vi "Write Sweep Rate (No Objects).vi"(8 "error in (no error)":errorcluster, 10 "rate":dbl[unit] caption="Rate", 11 "Cluster In":T4={"Field"=0.0, "Rate"=0.0, "Status"={"Sweeping"=FALSE, "Clamped"=FALSE, "Hold"=FALSE, "At Rest"=FALSE, "Quench"=FALSE, "Persistent Mode"=FALSE, "Switch Heater"=FALSE}, "ILM Shut Down?"=FALSE, "IO Info"={"Address"={"Com Port"=1, "ISOBUS Address"=2, "GPIB Address"=24, "Communication"=enum."ISOBUS"}, "Version"=enum."IPS"}, "IO Info (Level Meter)"={"Address"={"Com Port"=1, "ISOBUS Address"=5, "GPIB Address"=24, "Communication"=enum."ISOBUS"}, "ILM Name"="", "Display Channel"=[]}, "Training?"=FALSE, "Training Field and Speed Cluster"={"Training Field"=[0.0, 4.108, 5.78, 8.001], "Training Speed"=[0.0057, 0.0022833333333333334, 0.0011333333333333334, 0.0011333333333333334]}}) -> (0 "error out":errorcluster, 3 "Cluster Out":T4={"Field"=0.0, "Rate"=0.0, "Status"={"Sweeping"=FALSE, "Clamped"=FALSE, "Hold"=FALSE, "At Rest"=FALSE, "Quench"=FALSE, "Persistent Mode"=FALSE, "Switch Heater"=FALSE}, "ILM Shut Down?"=FALSE, "IO Info"={"Address"={"Com Port"=1, "ISOBUS Address"=2, "GPIB Address"=24, "Communication"=enum."ISOBUS"}, "Version"=enum."IPS"}, "IO Info (Level Meter)"={"Address"={"Com Port"=1, "ISOBUS Address"=5, "GPIB Address"=24, "Communication"=enum."ISOBUS"}, "ILM Name"="", "Display Channel"=[]}, "Training?"=FALSE, "Training Field and Speed Cluster"={"Training Field"=[0.0, 4.108, 5.78, 8.001], "Training Speed"=[0.0057, 0.0022833333333333334, 0.0011333333333333334, 0.0011333333333333334]}})   [LabVIEW 2017]
uses:
  Magnet status.ctl
  Oxford/PSSUBS.LLB/PSIO.ctl
  Oxford/BUSGEN.LLB/OxfordAddress.ctl
  Power Supply.lvclass
panel:
  out "rateok":bool
  out "maxrate":dbl[unit]
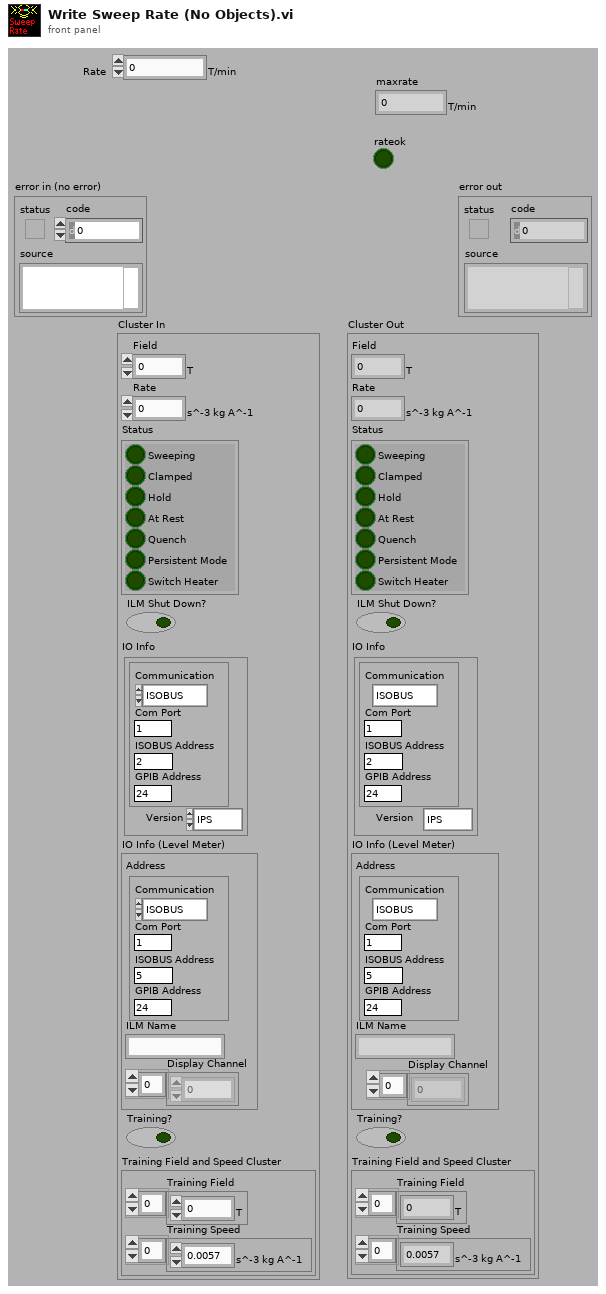
[diagram p1: front panel]
types:
  T1 = typedef "Power Supply.lvclass/Magnet status.ctl" = cluster{"Sweeping":bool, "Clamped":bool, "Hold":bool, "At Rest":bool, "Quench":bool, "Persistent Mode":bool, "Switch Heater":bool}
  T2 = typedef "PSIO.ctl" = cluster{"Address":T3, "Version":enum16{"PS", "IPS"}}
  T3 = typedef "OxfordAddress.ctl" = cluster{"Com Port":i32, "ISOBUS Address":i32, "GPIB Address":i16, "Communication":enum16{"RS232", "ISOBUS", "GPIB", "Gateway"}}
  T4 = cluster{"Field":dbl[unit], "Rate":dbl[unit], "Status":T1, "ILM Shut Down?":bool, "IO Info":T2, "IO Info (Level Meter)":cluster{"Address":T3, "ILM Name":string, "Display Channel":i32[]}, "Training?":bool, "Training Field and Speed Cluster":cluster{"Training Field":dbl[unit][], "Training Speed":dbl[unit][]}}
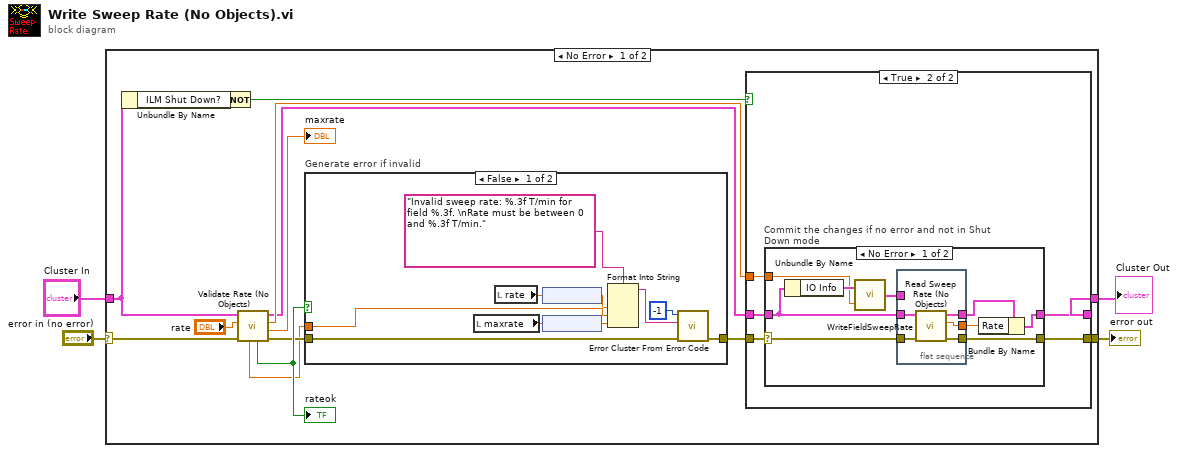
[diagram p0: block diagram]
diagram:
  n1 = case shown="No Error" "error in (no error)" {
    selector: "error in (no error)" -> [w14 w53]
    tunnel: [w18 w54] -> w2
    tunnel: [w15 w53] -> w3
    tunnel: "Cluster In" -> [w5 w54]
    frame No Error {
      n2 = Unbundle By Name(w5) -> ("ILM Shut Down?"=w7:bool)
      n3 = Not(x=w7) -> (.not. x?=w6:bool)
      n4 = call "Validate Rate (No Objects).vi"("error IO"=w14, "rate"="rate", "Cluster In"=w5) -> ("error out"=w13:errorcluster, "Max rate"=→"maxrate":dbl[unit], "Coerced rate"=w9:dbl[unit], "Cluster Out"=w8:T4, "Coerced?"=w16:bool, "Field"=w12:dbl[unit])  [unwired: 3 in]
      "rateok" <- w16
      n5 = case "Generate error if invalid" shown="False" w16 {
        tunnel: [w51 w52] -> w17
        tunnel: w13 -> [w47 w52]
        tunnel: w12 -> [w45 _]
        frame False {
          n6 = local read "maxrate"() -> (w46:dbl[unit])
          n7 = local read "rate"() -> (w44:dbl[unit])
          n8 = node(w44) -> (w43:dbl)
          n9 = node(w46) -> (w42:dbl)
          n10 = Format Into String(format string="Invalid sweep rate: %.3f T/min for field %.3f. \nRate must be between 0 and %.3f T/min.", w43, w45, w42) -> (resulting string=w49:string)  [unwired: 2 in, 1 out]
          n11 = call <vilib>:"Error Cluster From Error Code.vi"("error in (no error)"=w47, "error message (\"\")"=w49, "error code (0)"=-1) -> ("error out"=w51:errorcluster)  [unwired: 6 in]
        }
        frame True {
        }
      }
      n12 = case shown="True" w6 {
        tunnel: [w20 w25] -> w18
        tunnel: w17 -> [w19 w24]
        tunnel: [w19 w23] -> w15
        tunnel: w9 -> [_ w22]
        tunnel: w8 -> [w20 w21]
        frame False {
        }
        frame True {
          n13 = case "Commit the changes if no error and not in Shut Down mode" shown="No Error" w24 {
            selector: w24 -> [w27 w41]
            tunnel: w22 -> [w32 _]
            tunnel: [w26 w41] -> w23
            tunnel: w21 -> [w30 w40]
            tunnel: [w33 w40] -> w25
            frame No Error {
              n14 = Unbundle By Name(w30) -> ("IO Info"=w34:T2)
              n15 = call "WriteFieldSweepRate.vi"("Sweep rate"=w32, "IO Info"=w34) -> ("IO Info"=w28:T2)
              n16 = flat-sequence {
                tunnel: [w39] -> w31
                tunnel: w30 -> [w35]
                tunnel: [w38] -> w29
                tunnel: w28 -> [_]
                tunnel: w27 -> [w37]
                tunnel: [w36] -> w26
                frame #0 {
                  n17 = call "Read Sweep Rate (No Objects).vi"("error in (no error)"=w37, "Cluster In"=w35) -> ("error out"=w36:errorcluster, "Field sweep rate"=w39:dbl[unit], "Cluster Out"=w38:T4)  [unwired: 7 in]
                }
              }
              n18 = Bundle By Name(cluster=w29, "Rate"=w31) -> (w33:T4)
            }
            frame Error {
            }
          }
        }
      }
    }
    frame Error {
    }
  }
  "error out" <- w3
  "Cluster Out" <- w2
